vi "create_LS370_Data_header.vi"() -> (3 "String":string)   [LabVIEW 2016]
uses:
  Instrument_Setup.vi
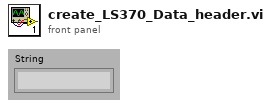
[diagram p1: front panel]
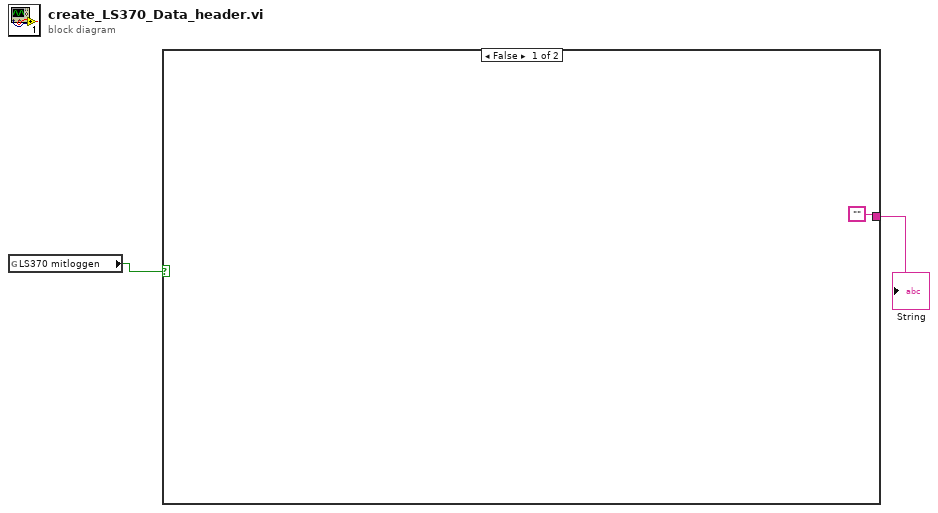
[diagram p0: block diagram]
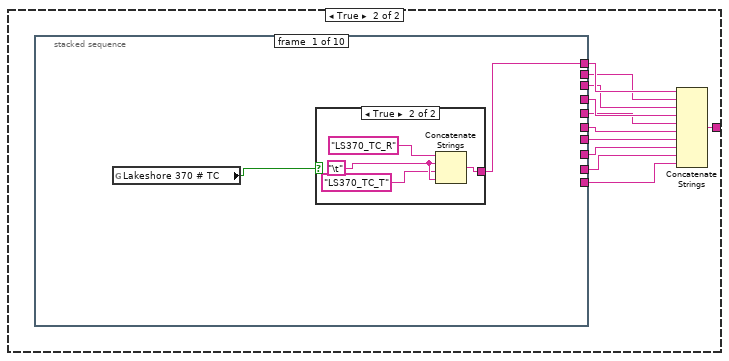
[diagram p2: hidden frame]
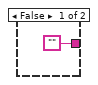
[diagram p3: hidden frame]
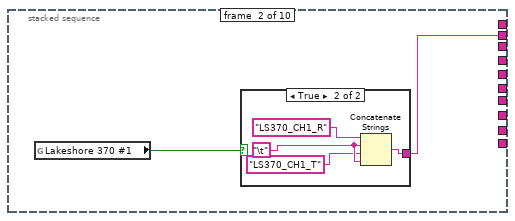
[diagram p4: hidden frame]
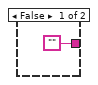
[diagram p5: hidden frame]
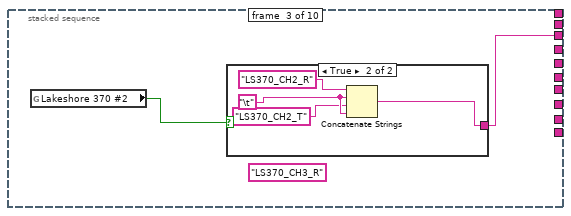
[diagram p6: hidden frame]
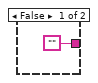
[diagram p7: hidden frame]
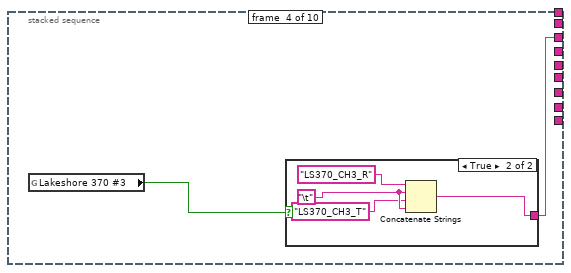
[diagram p8: hidden frame]
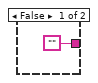
[diagram p9: hidden frame]
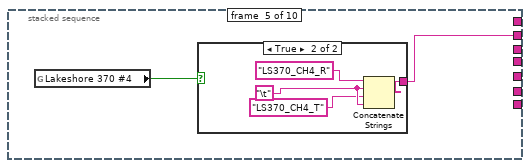
[diagram p10: hidden frame]
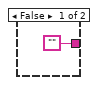
[diagram p11: hidden frame]
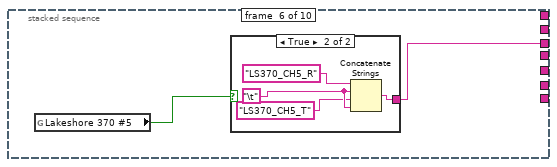
[diagram p12: hidden frame]
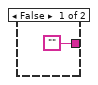
[diagram p13: hidden frame]
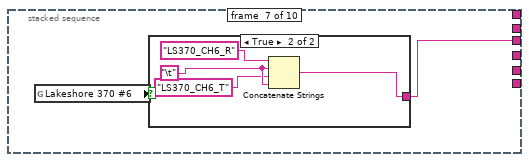
[diagram p14: hidden frame]
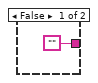
[diagram p15: hidden frame]
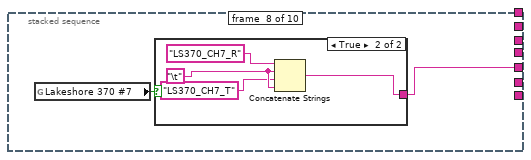
[diagram p16: hidden frame]
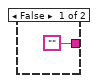
[diagram p17: hidden frame]
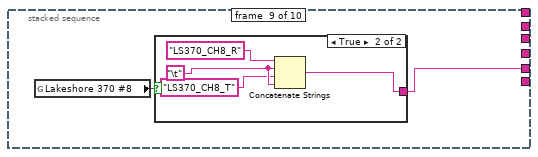
[diagram p18: hidden frame]
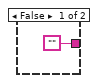
[diagram p19: hidden frame]
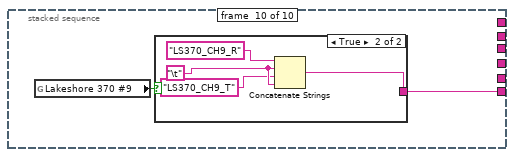
[diagram p20: hidden frame]
diagram:
  n1 = global read "Instrument_Setup.vi" "LS370 mitloggen"() -> (w1:bool)
  n2 = case shown="False" w1 {
    tunnel: ["" w4] -> w2
    frame False {
    }
    frame True {
      n3 = stacked-sequence {
        tunnel: [w15 _ _ _ _ _ _ _ _ _] -> w14
        tunnel: [_ w22 _ _ _ _ _ _ _ _] -> w13
        tunnel: [_ _ w29 _ _ _ _ _ _ _] -> w12
        tunnel: [_ _ _ w36 _ _ _ _ _ _] -> w11
        tunnel: [_ _ _ _ w43 _ _ _ _ _] -> w10
        tunnel: [_ _ _ _ _ w50 _ _ _ _] -> w9
        tunnel: [_ _ _ _ _ _ w57 _ _ _] -> w8
        tunnel: [_ _ _ _ _ _ _ w64 _ _] -> w7
        tunnel: [_ _ _ _ _ _ _ _ w71 _] -> w6
        tunnel: [_ _ _ _ _ _ _ _ _ w78] -> w5
        frame #0 {
          n4 = global read "Instrument_Setup.vi" "Lakeshore 370 # TC"() -> (w16:bool)
          n5 = case shown="True" w16 {
            tunnel: ["" w21] -> w15
            frame False {
            }
            frame True {
              w19 = "\t"
              n6 = Concatenate Strings("LS370_TC_R", w19, "LS370_TC_T", w19) -> (w21:string)
            }
          }
        }
        frame #1 {
          n7 = global read "Instrument_Setup.vi" "Lakeshore 370 #1"() -> (w23:bool)
          n8 = case shown="True" w23 {
            tunnel: ["" w28] -> w22
            frame False {
            }
            frame True {
              w26 = "\t"
              n9 = Concatenate Strings("LS370_CH1_R", w26, "LS370_CH1_T", w26) -> (w28:string)
            }
          }
        }
        frame #2 {
          (unwired) "LS370_CH3_R"
          n10 = global read "Instrument_Setup.vi" "Lakeshore 370 #2"() -> (w30:bool)
          n11 = case shown="True" w30 {
            tunnel: ["" w32] -> w29
            frame False {
            }
            frame True {
              w34 = "\t"
              n12 = Concatenate Strings("LS370_CH2_R", w34, "LS370_CH2_T", w34) -> (w32:string)
            }
          }
        }
        frame #3 {
          n13 = global read "Instrument_Setup.vi" "Lakeshore 370 #3"() -> (w37:bool)
          n14 = case shown="True" w37 {
            tunnel: ["" w39] -> w36
            frame False {
            }
            frame True {
              w41 = "\t"
              n15 = Concatenate Strings("LS370_CH3_R", w41, "LS370_CH3_T", w41) -> (w39:string)
            }
          }
        }
        frame #4 {
          n16 = global read "Instrument_Setup.vi" "Lakeshore 370 #4"() -> (w44:bool)
          n17 = case shown="True" w44 {
            tunnel: ["" w46] -> w43
            frame False {
            }
            frame True {
              w48 = "\t"
              n18 = Concatenate Strings("LS370_CH4_R", w48, "LS370_CH4_T", w48) -> (w46:string)
            }
          }
        }
        frame #5 {
          n19 = global read "Instrument_Setup.vi" "Lakeshore 370 #5"() -> (w51:bool)
          n20 = case shown="True" w51 {
            tunnel: ["" w53] -> w50
            frame False {
            }
            frame True {
              w55 = "\t"
              n21 = Concatenate Strings("LS370_CH5_R", w55, "LS370_CH5_T", w55) -> (w53:string)
            }
          }
        }
        frame #6 {
          n22 = global read "Instrument_Setup.vi" "Lakeshore 370 #6"() -> (w58:bool)
          n23 = case shown="True" w58 {
            tunnel: ["" w60] -> w57
            frame False {
            }
            frame True {
              w62 = "\t"
              n24 = Concatenate Strings("LS370_CH6_R", w62, "LS370_CH6_T", w62) -> (w60:string)
            }
          }
        }
        frame #7 {
          n25 = global read "Instrument_Setup.vi" "Lakeshore 370 #7"() -> (w65:bool)
          n26 = case shown="True" w65 {
            tunnel: ["" w67] -> w64
            frame False {
            }
            frame True {
              w69 = "\t"
              n27 = Concatenate Strings("LS370_CH7_R", w69, "LS370_CH7_T", w69) -> (w67:string)
            }
          }
        }
        frame #8 {
          n28 = global read "Instrument_Setup.vi" "Lakeshore 370 #8"() -> (w72:bool)
          n29 = case shown="True" w72 {
            tunnel: ["" w74] -> w71
            frame False {
            }
            frame True {
              w76 = "\t"
              n30 = Concatenate Strings("LS370_CH8_R", w76, "LS370_CH8_T", w76) -> (w74:string)
            }
          }
        }
        frame #9 {
          n31 = global read "Instrument_Setup.vi" "Lakeshore 370 #9"() -> (w79:bool)
          n32 = case shown="True" w79 {
            tunnel: ["" w81] -> w78
            frame False {
            }
            frame True {
              w83 = "\t"
              n33 = Concatenate Strings("LS370_CH9_R", w83, "LS370_CH9_T", w83) -> (w81:string)
            }
          }
        }
      }
      n34 = Concatenate Strings(w14, w13, w12, w11, w10, w9, w8, w7, w6, w5) -> (w4:string)
    }
  }
  "String" <- w2
